vi "delete sequence.vi"(8 "error in (no error)":errorcluster, 10 "sequence name":string, 11 "Simple Sequencer TBM configuration in":refnum<class "Simple Sequencer TBM configuration.lvclass">) -> (0 "error out":errorcluster, 3 "Simple Sequencer TBM configuration out":refnum<class "Simple Sequencer TBM configuration.lvclass">)   [LabVIEW 2014, in "Simple Sequencer TBM configuration.lvclass"]
doc: "Removes the sequence of the specified name."
uses:
  Simple Sequencer TBM configuration.lvclass
  Simple Sequencer TBM configuration.lvclass/Simple Sequencer TBM configuration.ctl
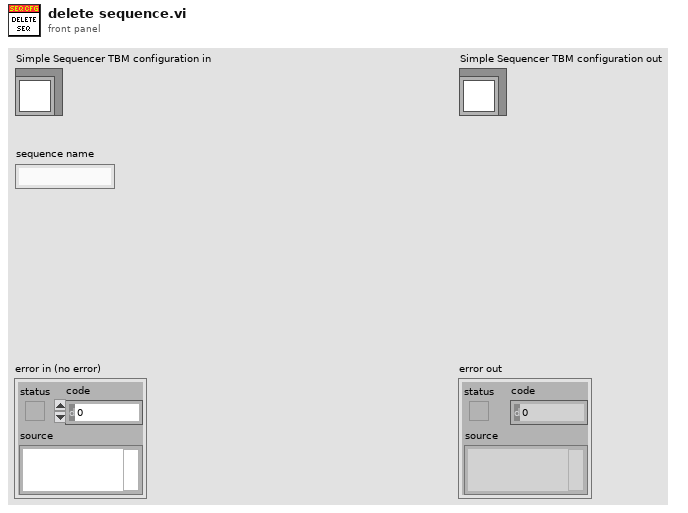
[diagram p1: front panel]
types:
  T1 = typedef "Simple Sequencer TBM configuration.lvclass/sequence definition.ctl" = cluster{"sequence name":string, "action configs":refnum<class "action configuration.lvclass">[]}
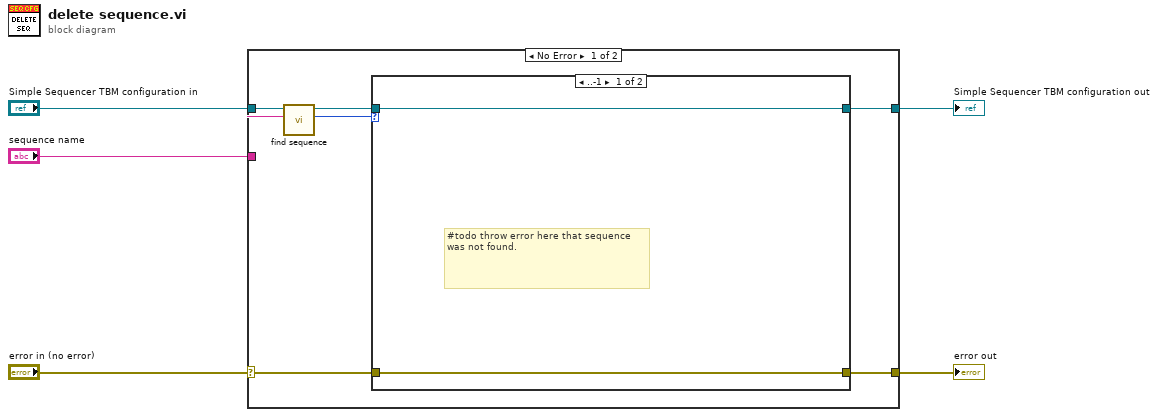
[diagram p0: block diagram]
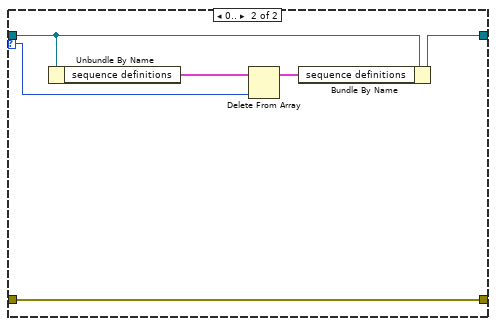
[diagram p2: hidden frame]
diagram:
  n1 = case shown="No Error" "error in (no error)" {
    selector: "error in (no error)" -> [w10 w22]
    tunnel: [w11 w22] -> w4
    tunnel: [w12 w21] -> w2
    tunnel: "Simple Sequencer TBM configuration in" -> [w9 w21]
    tunnel: "sequence name" -> [w7 _]
    frame No Error {
      n2 = call "find sequence.vi"("sequence name"=w7, "Simple Sequencer TBM configuration in"=w9) -> ("index"=w6:i32, "Simple Sequencer TBM configuration out"=w8:refnum<class "Simple Sequencer TBM configuration.lvclass">)  [unwired: 8 in]
      n3 = case shown="..-1" w6 {
        selector: w6 -> [_ w15]
        tunnel: w8 -> [w14 w17]
        tunnel: [w14 w18] -> w12
        tunnel: [w13 w20] -> w11
        tunnel: w10 -> [w13 w20]
        frame ..-1 {
          # "#todo throw error here that sequence\nwas not found."
        }
        frame 0.. {
          n4 = Unbundle By Name(w17) -> ("sequence definitions"=w16:T1[])
          n5 = Delete From Array(array=w16, index=w15) -> (array with subset deleted=w19:T1[])  [unwired: 1 in, 1 out]
          n6 = Bundle By Name(cluster=w17, "sequence definitions"=w19) -> (w18:refnum<class "Simple Sequencer TBM configuration.lvclass">)
        }
      }
    }
    frame Error {
    }
  }
  "error out" <- w4
  "Simple Sequencer TBM configuration out" <- w2
